vi "Detect TSw.vi"(9 "Side Gyro Data":T1={"Time"=0.0, "Gyro Array Data"=[], "Gyro Negation"=[], "Gyro Data"={"Gyro X"=0.0, "Gyro Y"=0.0, "Gyro Z"=0.0}, "Gyro Latency"=0.0, "Normalization Time"=640.0, "Sampling Rate"=0.0}, 10 "Side Event Data":T3={"Event Data"={"LR"={"Phase"="LR", "On"=FALSE, "Last On Time"=0.0, "Duration"=0.0, "Crossing Time"=0.0, "Time since LR"=0.0, "Time Since TSw"=0.0, "Min gyro Z"=0.0, "Time since LR?"=FALSE, "Time since TSw?"=FALSE, "Min gyro Z?"=FALSE, "Crossing?"=FALSE}, "MSt"={"Phase"="MSt", "On"=FALSE, "Last On Time"=0.0, "Duration"=0.0}, "TSt"={"Phase"="TSt", "On"=FALSE, "Last On Time"=0.0, "Duration"=0.0}, "PSw"={"Phase"="PSw", "On"=FALSE, "Last On Time"=0.0, "Duration"=0.0}, "ISw"={"Phase"="ISw", "On"=FALSE, "Last On Time"=0.0, "Duration"=0.0, "Peak Time"=0.0, "Time since LR"=0.0, "Time since ISw"=0.0, "Time since LR?"=FALSE, "Time since ISw?"=FALSE, "Peak?"=FALSE}, "MSw"={"Phase"="MSw", "On"=FALSE, "Last On Time"=0.0, "Duration"=0.0, "Crossing time"=0.0, "Time since LR"=0.0, "Time since MSw"=0.0, "Time since ISw"=0.0, "Time since LR?"=FALSE, "Time since MSw?"=FALSE, "Time since ISw?"=FALSE, "Crossing?"=FALSE}, "TSw"={"Phase"="TSw", "On"=FALSE, "Last On Time"=0.0, "Duration"=0.0, "Peak time"=0.0, "Time since LR"=0.0, "Time since TSw"=0.0, "Time since LR?"=FALSE, "Time since TSw?"=FALSE, "Peak?"=FALSE}}, "Mean Cycle Duration"=0.0, "Event Detected?"=FALSE, "Last Event Detected"=0, "Num Cycles"=0.0, "GPD Log"=refnum, "Last Event Time"=0.0}, 11 "GPD Parameters":T4={"% Cycle Delay"=0.0, "Min % Cycle LR to ISw "=0.0, "Min % Cycle LR to MSw"=0.0, "Min % Cycle LR to TSw"=0.0, "Max % Cycle ISw to MSw"=0.0, "Min % Cycle TSw to LR"=0.0, "Max % Cycle TSw to LR"=0.0, "LR Min Gyro Z Threshold"=0.0, "LR Min Gyro Z Width"=0.0, "ISw Peak Threshold"=0.0, "ISw Peak Width"=0.0, "TSw Valley Threshold"=0.0, "TSw Valley Width (ms)"=7.0, "Max Cycle Time (s)"=0.0, "Mean Computation Window"=0.0, "CP subject?"=FALSE}) -> (1 "Side Gyro Data":T1={"Time"=0.0, "Gyro Array Data"=[], "Gyro Negation"=[], "Gyro Data"={"Gyro X"=0.0, "Gyro Y"=0.0, "Gyro Z"=0.0}, "Gyro Latency"=0.0, "Normalization Time"=640.0, "Sampling Rate"=0.0}, 2 "Side Event Data":T3={"Event Data"={"LR"={"Phase"="LR", "On"=FALSE, "Last On Time"=0.0, "Duration"=0.0, "Crossing Time"=0.0, "Time since LR"=0.0, "Time Since TSw"=0.0, "Min gyro Z"=0.0, "Time since LR?"=FALSE, "Time since TSw?"=FALSE, "Min gyro Z?"=FALSE, "Crossing?"=FALSE}, "MSt"={"Phase"="MSt", "On"=FALSE, "Last On Time"=0.0, "Duration"=0.0}, "TSt"={"Phase"="TSt", "On"=FALSE, "Last On Time"=0.0, "Duration"=0.0}, "PSw"={"Phase"="PSw", "On"=FALSE, "Last On Time"=0.0, "Duration"=0.0}, "ISw"={"Phase"="ISw", "On"=FALSE, "Last On Time"=0.0, "Duration"=0.0, "Peak Time"=0.0, "Time since LR"=0.0, "Time since ISw"=0.0, "Time since LR?"=FALSE, "Time since ISw?"=FALSE, "Peak?"=FALSE}, "MSw"={"Phase"="MSw", "On"=FALSE, "Last On Time"=0.0, "Duration"=0.0, "Crossing time"=0.0, "Time since LR"=0.0, "Time since MSw"=0.0, "Time since ISw"=0.0, "Time since LR?"=FALSE, "Time since MSw?"=FALSE, "Time since ISw?"=FALSE, "Crossing?"=FALSE}, "TSw"={"Phase"="TSw", "On"=FALSE, "Last On Time"=0.0, "Duration"=0.0, "Peak time"=0.0, "Time since LR"=0.0, "Time since TSw"=0.0, "Time since LR?"=FALSE, "Time since TSw?"=FALSE, "Peak?"=FALSE}}, "Mean Cycle Duration"=0.0, "Event Detected?"=FALSE, "Last Event Detected"=0, "Num Cycles"=0.0, "GPD Log"=refnum, "Last Event Time"=0.0}, 3 "GPD Parameters out":T4={"% Cycle Delay"=0.0, "Min % Cycle LR to ISw "=0.0, "Min % Cycle LR to MSw"=0.0, "Min % Cycle LR to TSw"=0.0, "Max % Cycle ISw to MSw"=0.0, "Min % Cycle TSw to LR"=0.0, "Max % Cycle TSw to LR"=0.0, "LR Min Gyro Z Threshold"=0.0, "LR Min Gyro Z Width"=0.0, "ISw Peak Threshold"=0.0, "ISw Peak Width"=0.0, "TSw Valley Threshold"=0.0, "TSw Valley Width (ms)"=7.0, "Max Cycle Time (s)"=0.0, "Mean Computation Window"=0.0, "CP subject?"=FALSE}, 4 "TSW Detected?":bool)   [LabVIEW 2019]
uses:
  Controls/GPD Side Parameters.ctl
  Controls/Side Event Data.ctl
  Controls/Gyro Side Data.ctl
  Controls/Gyro Negation.ctl
  <vilib>/ptbypt/NI_PtbyPt.lvlib
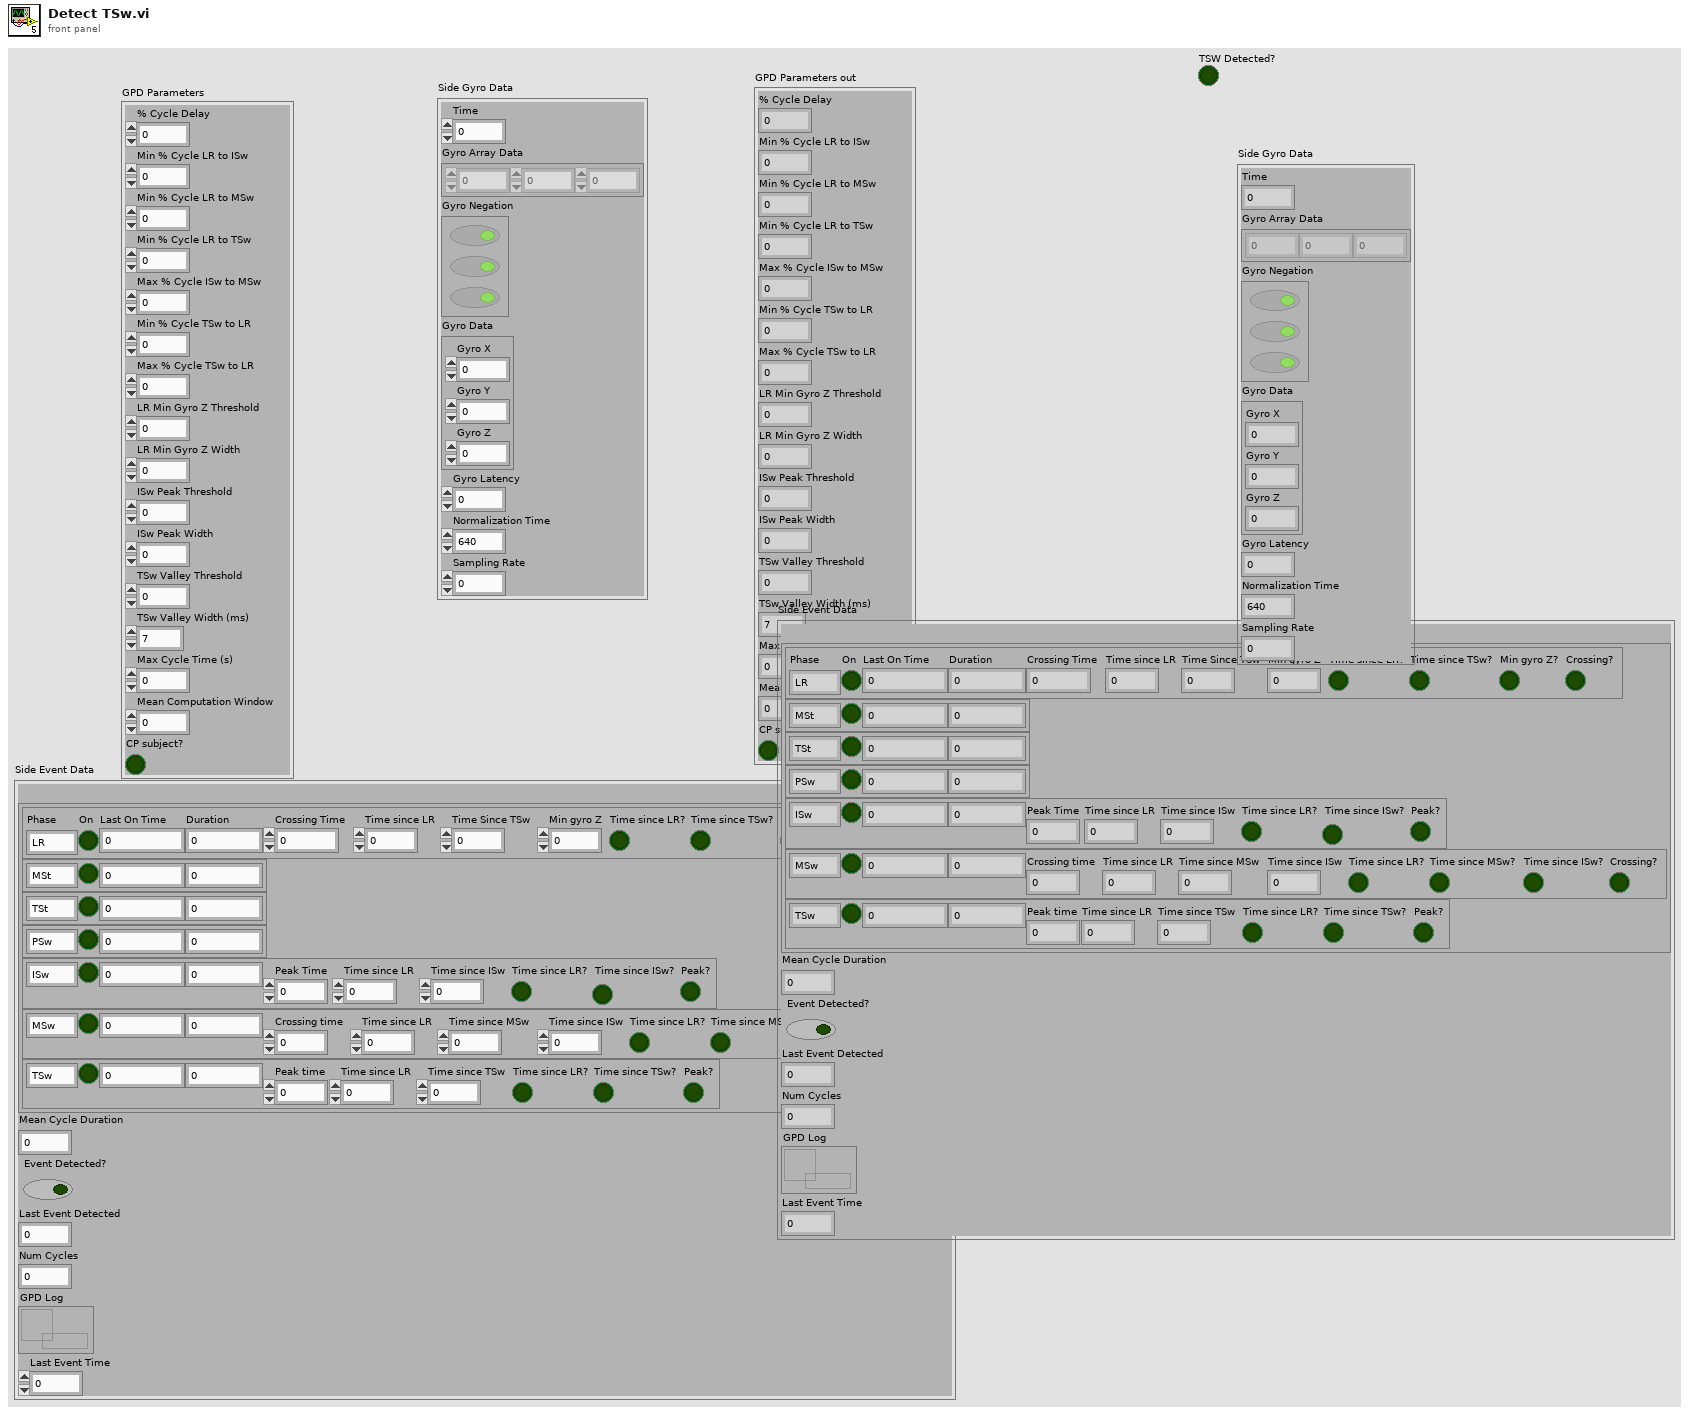
[diagram p1: front panel]
types:
  T1 = typedef "Gyro Side Data.ctl" = cluster{"Time":dbl, "Gyro Array Data":dbl[], "Gyro Negation":T2, "Gyro Data":cluster{"Gyro X":dbl, "Gyro Y":dbl, "Gyro Z":dbl}, "Gyro Latency":dbl, "Normalization Time":dbl, "Sampling Rate":dbl}
  T2 = typedef "Gyro Negation.ctl" = bool[]
  T3 = typedef "Side Event Data.ctl" = cluster{"Event Data":cluster{"LR":cluster{"Phase":string, "On":bool, "Last On Time":dbl, "Duration":dbl, "Crossing Time":dbl, "Time since LR":dbl, "Time Since TSw":dbl, "Min gyro Z":dbl, "Time since LR?":bool, "Time since TSw?":bool, "Min gyro Z?":bool, "Crossing?":bool}, "MSt":cluster{"Phase":string, "On":bool, "Last On Time":dbl, "Duration":dbl}, "TSt":cluster{"Phase":string, "On":bool, "Last On Time":dbl, "Duration":dbl}, "PSw":cluster{"Phase":string, "On":bool, "Last On Time":dbl, "Duration":dbl}, "ISw":cluster{"Phase":string, "On":bool, "Last On Time":dbl, "Duration":dbl, "Peak Time":dbl, "Time since LR":dbl, "Time since ISw":dbl, "Time since LR?":bool, "Time since ISw?":bool, "Peak?":bool}, "MSw":cluster{"Phase":string, "On":bool, "Last On Time":dbl, "Duration":dbl, "Crossing time":dbl, "Time since LR":dbl, "Time since MSw":dbl, "Time since ISw":dbl, "Time since LR?":bool, "Time since MSw?":bool, "Time since ISw?":bool, "Crossing?":bool}, "TSw":cluster{"Phase":string, "On":bool, "Last On Time":dbl, "Duration":dbl, "Peak time":dbl, "Time since LR":dbl, "Time since TSw":dbl, "Time since LR?":bool, "Time since TSw?":bool, "Peak?":bool}}, "Mean Cycle Duration":dbl, "Event Detected?":bool, "Last Event Detected":i32, "Num Cycles":dbl, "GPD Log":refnum<queue>, "Last Event Time":dbl}
  T4 = typedef "GPD Side Parameters.ctl" = cluster{"% Cycle Delay":dbl, "Min % Cycle LR to ISw ":dbl, "Min % Cycle LR to MSw":dbl, "Min % Cycle LR to TSw":dbl, "Max % Cycle ISw to MSw":dbl, "Min % Cycle TSw to LR":dbl, "Max % Cycle TSw to LR":dbl, "LR Min Gyro Z Threshold":dbl, "LR Min Gyro Z Width":dbl, "ISw Peak Threshold":dbl, "ISw Peak Width":dbl, "TSw Valley Threshold":dbl, "TSw Valley Width (ms)":dbl, "Max Cycle Time (s)":dbl, "Mean Computation Window":dbl, "CP subject?":bool}
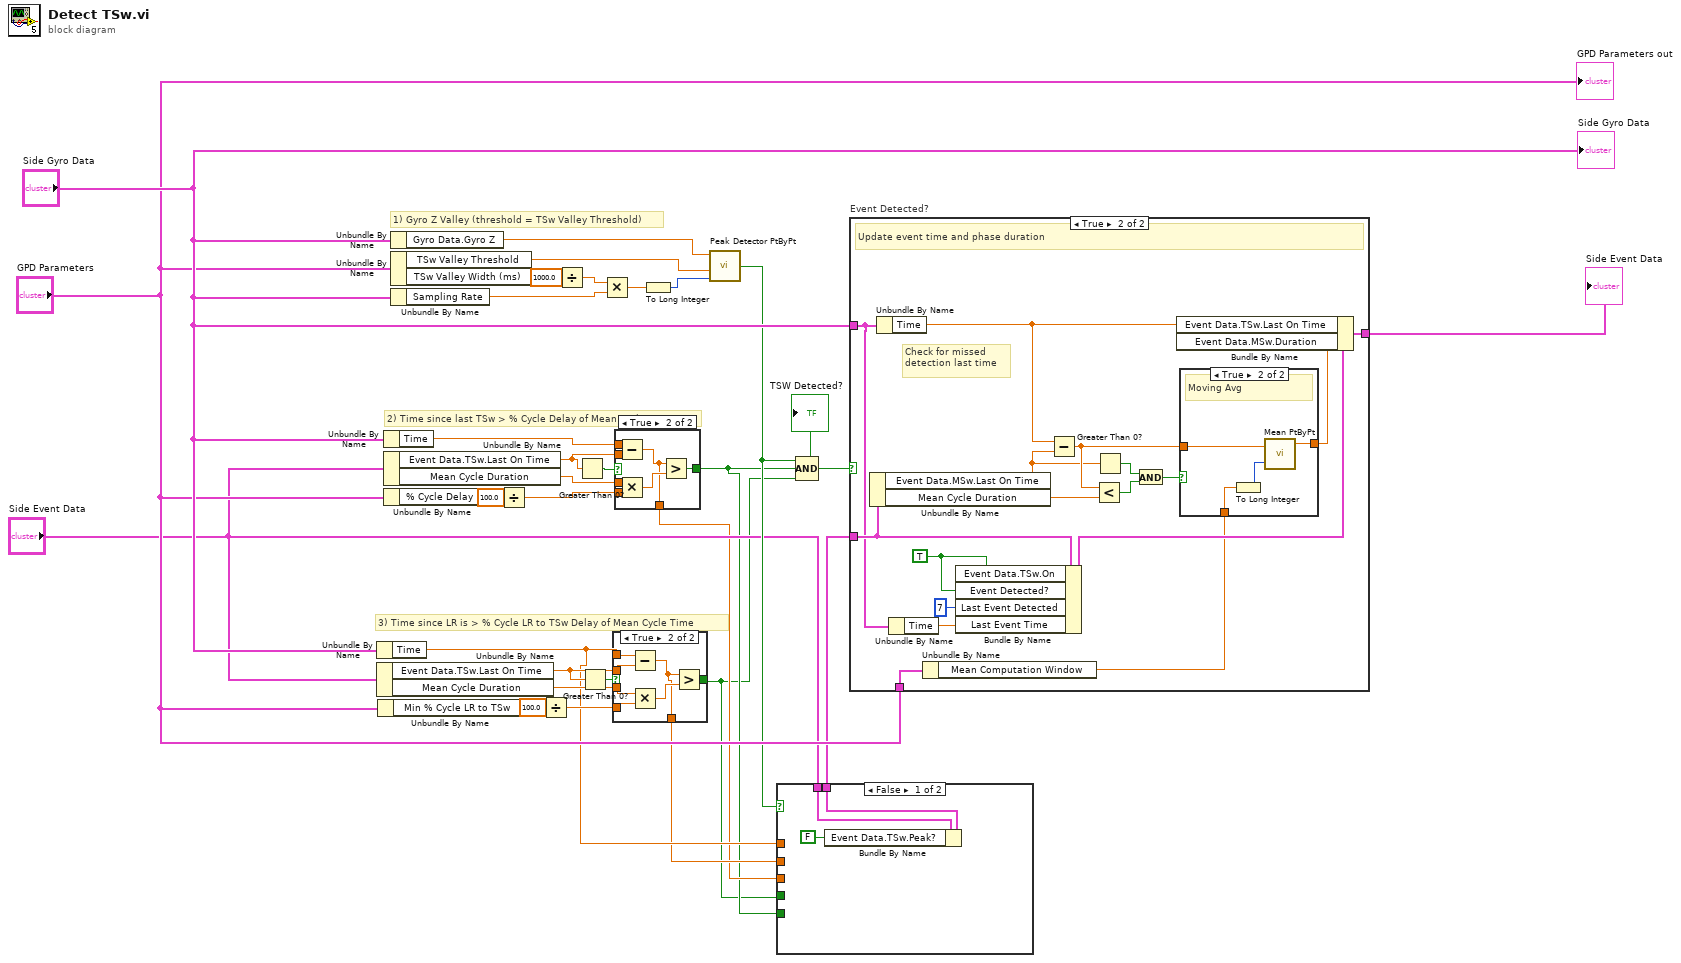
[diagram p0: block diagram]
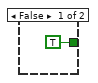
[diagram p2: hidden frame]
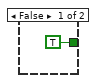
[diagram p3: hidden frame]
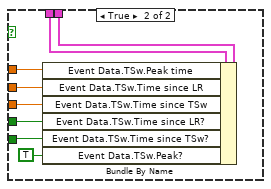
[diagram p4: hidden frame]
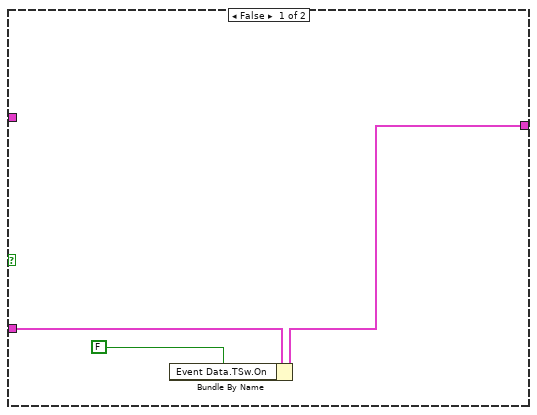
[diagram p5: hidden frame]
diagram:
  # "3) Time since LR is > % Cycle LR to TSw Delay of Mean Cycle Time"
  # "2) Time since last TSw > % Cycle Delay of Mean Cycle Time"
  # "1) Gyro Z Valley (threshold = TSw Valley Threshold)"
  n1 = Unbundle By Name("Side Gyro Data") -> ("Time"=w5:dbl)
  n2 = Unbundle By Name("Side Event Data") -> ("Event Data.TSw.Last On Time"=w9:dbl, "Mean Cycle Duration"=w19:dbl)
  n3 = Unbundle By Name("GPD Parameters") -> ("Min % Cycle LR to TSw"=w18:dbl)
  n4 = Unbundle By Name("Side Gyro Data") -> ("Time"=w24:dbl)
  n5 = Unbundle By Name("Side Event Data") -> ("Event Data.TSw.Last On Time"=w12:dbl, "Mean Cycle Duration"=w23:dbl)
  n6 = Unbundle By Name("GPD Parameters") -> ("% Cycle Delay"=w22:dbl)
  n7 = Unbundle By Name("Side Gyro Data") -> ("Gyro Data.Gyro Z"=w25:dbl)
  n8 = Unbundle By Name("GPD Parameters") -> ("TSw Valley Threshold"=w30:dbl, "TSw Valley Width (ms)"=w29:dbl)
  n9 = Unbundle By Name("Side Gyro Data") -> ("Sampling Rate"=w27:dbl)
  n10 = Divide(x=w22, y=100.0) -> (x/y=w20:dbl)
  n11 = Divide(x=w18, y=100.0) -> (x/y=w16:dbl)
  n12 = Divide(x=w29, y=1000.0) -> (x/y=w26:dbl)
  n13 = Greater Than 0?(x=w12) -> (x > 0?=w11:bool)
  n14 = Greater Than 0?(x=w9) -> (x > 0?=w10:bool)
  n15 = Multiply(x=w26, y=w27) -> (x*y=w31:dbl)
  n16 = case shown="True" w10 {
    tunnel: w5 -> [_ w41]
    tunnel: w9 -> [_ w40]
    tunnel: w19 -> [_ w39]
    tunnel: w16 -> [_ w37]
    tunnel: [TRUE w36] -> w1
    tunnel: [_ w35] -> w4
    frame False {
    }
    frame True {
      n17 = Subtract(x=w41, y=w40) -> (x-y=w35:dbl)
      n18 = Multiply(x=w39, y=w37) -> (x*y=w38:dbl)
      n19 = Greater?(x=w35, y=w38) -> (0:w36:bool)
    }
  }
  n20 = case shown="True" w11 {
    tunnel: w24 -> [_ w49]
    tunnel: w12 -> [_ w48]
    tunnel: w23 -> [_ w47]
    tunnel: w20 -> [_ w45]
    tunnel: [TRUE w44] -> w2
    tunnel: [_ w43] -> w3
    frame False {
    }
    frame True {
      n21 = Subtract(x=w49, y=w48) -> (x-y=w43:dbl)
      n22 = Multiply(x=w47, y=w45) -> (x*y=w46:dbl)
      n23 = Greater?(x=w43, y=w46) -> (0:w44:bool)
    }
  }
  n24 = To Long Integer(number=w31) -> (32bit integer=w32:i32)
  n25 = call <vilib>:"Peak Detector PtByPt.vi"("x"=w25, "threshold valley"=w30, "width"=w32) -> ("valley"=w8:bool)  [unwired: 2 in, 2 out]
  n26 = case shown="False" w8 {
    tunnel: "Side Event Data" -> [w51 w60]
    tunnel: [w50 w59] -> w6
    tunnel: w5 -> [_ w58]
    tunnel: w4 -> [_ w57]
    tunnel: w3 -> [_ w56]
    tunnel: w1 -> [_ w55]
    tunnel: w2 -> [_ w54]
    frame False {
      n27 = Bundle By Name(cluster=w51, "Event Data.TSw.Peak?"=FALSE) -> (w50:T3)
    }
    frame True {
      n28 = Bundle By Name(cluster=w60, "Event Data.TSw.Peak time"=w58, "Event Data.TSw.Time since LR"=w57, "Event Data.TSw.Time since TSw"=w56, "Event Data.TSw.Time since LR?"=w55, "Event Data.TSw.Time since TSw?"=w54, "Event Data.TSw.Peak?"=TRUE) -> (w59:T3)
    }
  }
  n29 = Compound Arithmetic op=AND(w8, w2, w1) -> (w15:bool)
  "TSW Detected?" <- w15
  n30 = case "Event Detected?" shown="True" w15 {
    tunnel: w6 -> [w62 w76]
    tunnel: [w61 w80] -> w33
    tunnel: "Side Gyro Data" -> [_ w64]
    tunnel: "GPD Parameters" -> [_ w71]
    frame False {
      n31 = Bundle By Name(cluster=w62, "Event Data.TSw.On"=FALSE) -> (w61:T3)
    }
    frame True {
      w74 = TRUE
      # "Check for missed detection last time"
      # "Update event time and phase duration"
      n32 = Unbundle By Name(w76) -> ("Event Data.MSw.Last On Time"=w69:dbl, "Mean Cycle Duration"=w79:dbl)
      n33 = Unbundle By Name(w64) -> ("Time"=w72:dbl)
      n34 = Unbundle By Name(w64) -> ("Time"=w65:dbl)
      n35 = Unbundle By Name(w71) -> ("Mean Computation Window"=w70:dbl)
      n36 = Bundle By Name(cluster=w76, "Event Data.TSw.On"=w74, "Event Detected?"=w74, "Last Event Detected"=7, "Last Event Time"=w65) -> (w75:T3)
      n37 = Subtract(x=w72, y=w69) -> (x-y=w78:dbl)
      n38 = Less?(x=w78, y=w79) -> (x < y?=w67:bool)
      n39 = Greater Than 0?(x=w69) -> (x > 0?=w68:bool)
      n40 = And(x=w68, y=w67) -> (x .and. y?=w66:bool)
      n41 = case shown="True" w66 {
        tunnel: w78 -> [w81 w85]
        tunnel: [w81 w84] -> w77
        tunnel: w70 -> [_ w82]
        frame False {
        }
        frame True {
          # "Moving Avg"
          n42 = To Long Integer(number=w82) -> (32bit integer=w83:i32)
          n43 = call <vilib>:"Mean PtByPt.vi"("x"=w85, "sample length"=w83) -> ("mean"=w84:dbl)  [unwired: 2 in, 1 out]
        }
      }
      n44 = Bundle By Name(cluster=w75, "Event Data.TSw.Last On Time"=w72, "Event Data.MSw.Duration"=w77) -> (w80:T3)
    }
  }
  "Side Event Data" <- w33
  "GPD Parameters out" <- "GPD Parameters"
  "Side Gyro Data" <- "Side Gyro Data"
